vi "Map.vi"() -> ()   [LabVIEW 2015]
uses:
  Robot.ctl
  Instruction.ctl
  class/Car.lvclass
  class/Instruction.lvclass
  class/MovementInstruction.lvclass
  class/TurnInstruction.lvclass
  class/StopInstruction.lvclass
  <vilib>/rvi/interface/nirviReadWriteControl/nirviReadWriteControl.xnode
  class/SonarSensor.lvclass
  <vilib>/rvi/interface/nirviCloseFPGA/nirviCloseFPGA.xnode
  <vilib>/rvi/interface/nirviOpenFPGA/nirviOpenFPGA.xnode
  NiFpgaLv.dll
  <vilib>/Utility/error.llb/Error Cluster From Error Code.vi
  <vilib>/rvi/interface/Simulation/niFpgaSimulationCallBeginRW.vi
  <vilib>/rvi/errors/niLvFpgaAdjustHostInterfaceError.vi
  <vilib>/FPGAPlugInAG/Dynamic/niLvFpga_Close_Dynamic.vi
  FPGA Bitfiles/Milestone4_FPGATarget_FPGAReadSonars_MhsUmP2nS8s.lvbitx
  physical_robot/FPGA Read Sonars.vi
  <vilib>/FPGAPlugInAG/myRIO-1900/niLvFpga_Open_myRIO-1900.vi
  <vilib>/rvi/interface/common/dynamic/niFpgaDynamicAddResources.vi
panel:
  out "millisecond timer value":u32
  out "x .or. y?":bool
  out "Sim Robot Properties":T1={"Position"=[0.0, 0.0], "Size"=50.0, "Facing"=0.0, "Movement Ratios"=[0.0, -1.0], "Wheel Angle"=0.0}
  in  "Robot Properties":T1={"Position"=[500.0, 500.0], "Size"=33.0, "Facing"=0.0, "Movement Ratios"=[0.0, -1.0], "Wheel Angle"=0.0}
  out "Completed":bool
  out "Instruction Number":i32
  in  "Instructions":T2[](array[typedef])=[{"Type"="Movement", "Variable A"=30.0, "Variable B"=300.0, "Variable C"=0.0}, {"Type"="Turn", "Variable A"=30.0, "Variable B"=20.0, "Variable C"=90.0}, {"Type"="Movement", "Variable A"=30.0, "Variable B"=250.0, "Variable C"=0.0}, {"Type"="Turn", "Variable A"=30.0, "Variable B"=20.0, "Variable C"=90.0}, {"Type"="Movement", "Variable A"=30.0, "Variable B"=300.0, "Variable C"=0.0}, {"Type"="Stop", "Variable A"=3000.0, "Variable B"=0.0, "Variable C"=0.0}, {"Type"="Movement", "Variable A"=30.0, "Variable B"=200.0, "Variable C"=0.0}, {"Type"="Turn", "Variable A"=30.0, "Variable B"=-20.0, "Variable C"=90.0}, {"Type"="Movement", "Variable A"=30.0, "Variable B"=250.0, "Variable C"=0.0}, {"Type"="Turn", "Variable A"=30.0, "Variable B"=-20.0, "Variable C"=90.0}, {"Type"="Movement", "Variable A"=30.0, "Variable B"=300.0, "Variable C"=0.0}, {"Type"="Stop", "Variable A"=3000.0, "Variable B"=0.0, "Variable C"=0.0}]
  out "Robot Properties Output":T1
  in  "stop":bool
  in  "Obstacles":dbl[][](array[numeric])=[[100.0, 100.0, 420.0, 110.0], [100.0, 100.0, 110.0, 300.0], [100.0, 290.0, 420.0, 300.0], [410.0, 100.0, 420.0, 300.0], [205.0, 190.0, 215.0, 300.0], [305.0, 190.0, 315.0, 300.0]]
  out "2D Picture":picture
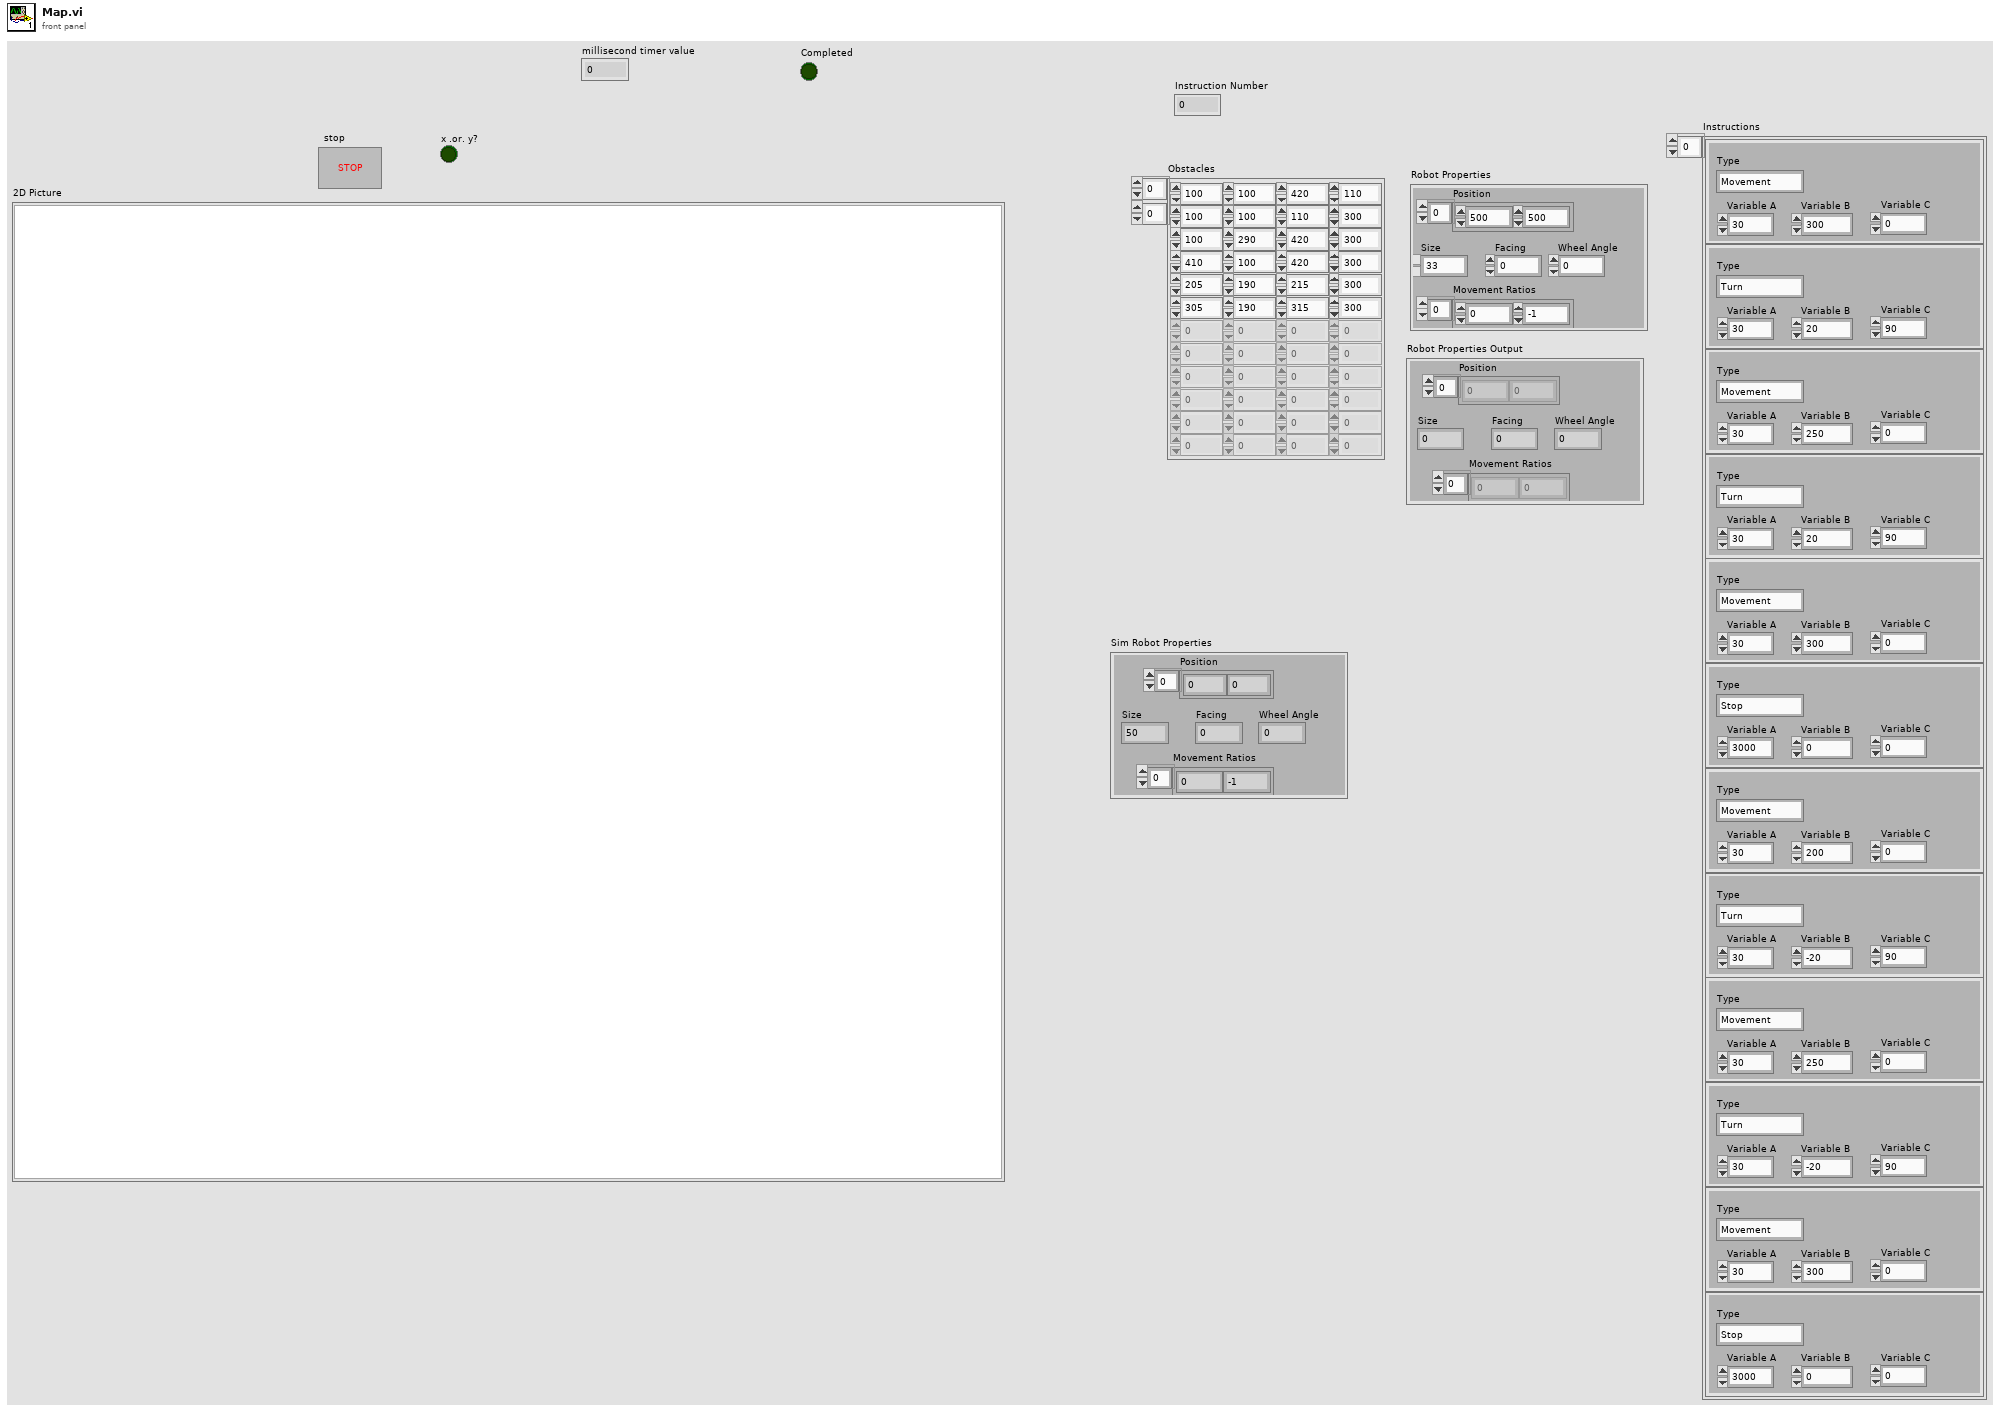
[diagram p1: front panel]
types:
  T1 = typedef "Robot.ctl" = cluster{"Position":dbl[], "Size":dbl, "Facing":dbl, "Movement Ratios":dbl[], "Wheel Angle":dbl}
  T2 = typedef "Instruction.ctl" = cluster{"Type":string, "Variable A":dbl, "Variable B":dbl, "Variable C":dbl}
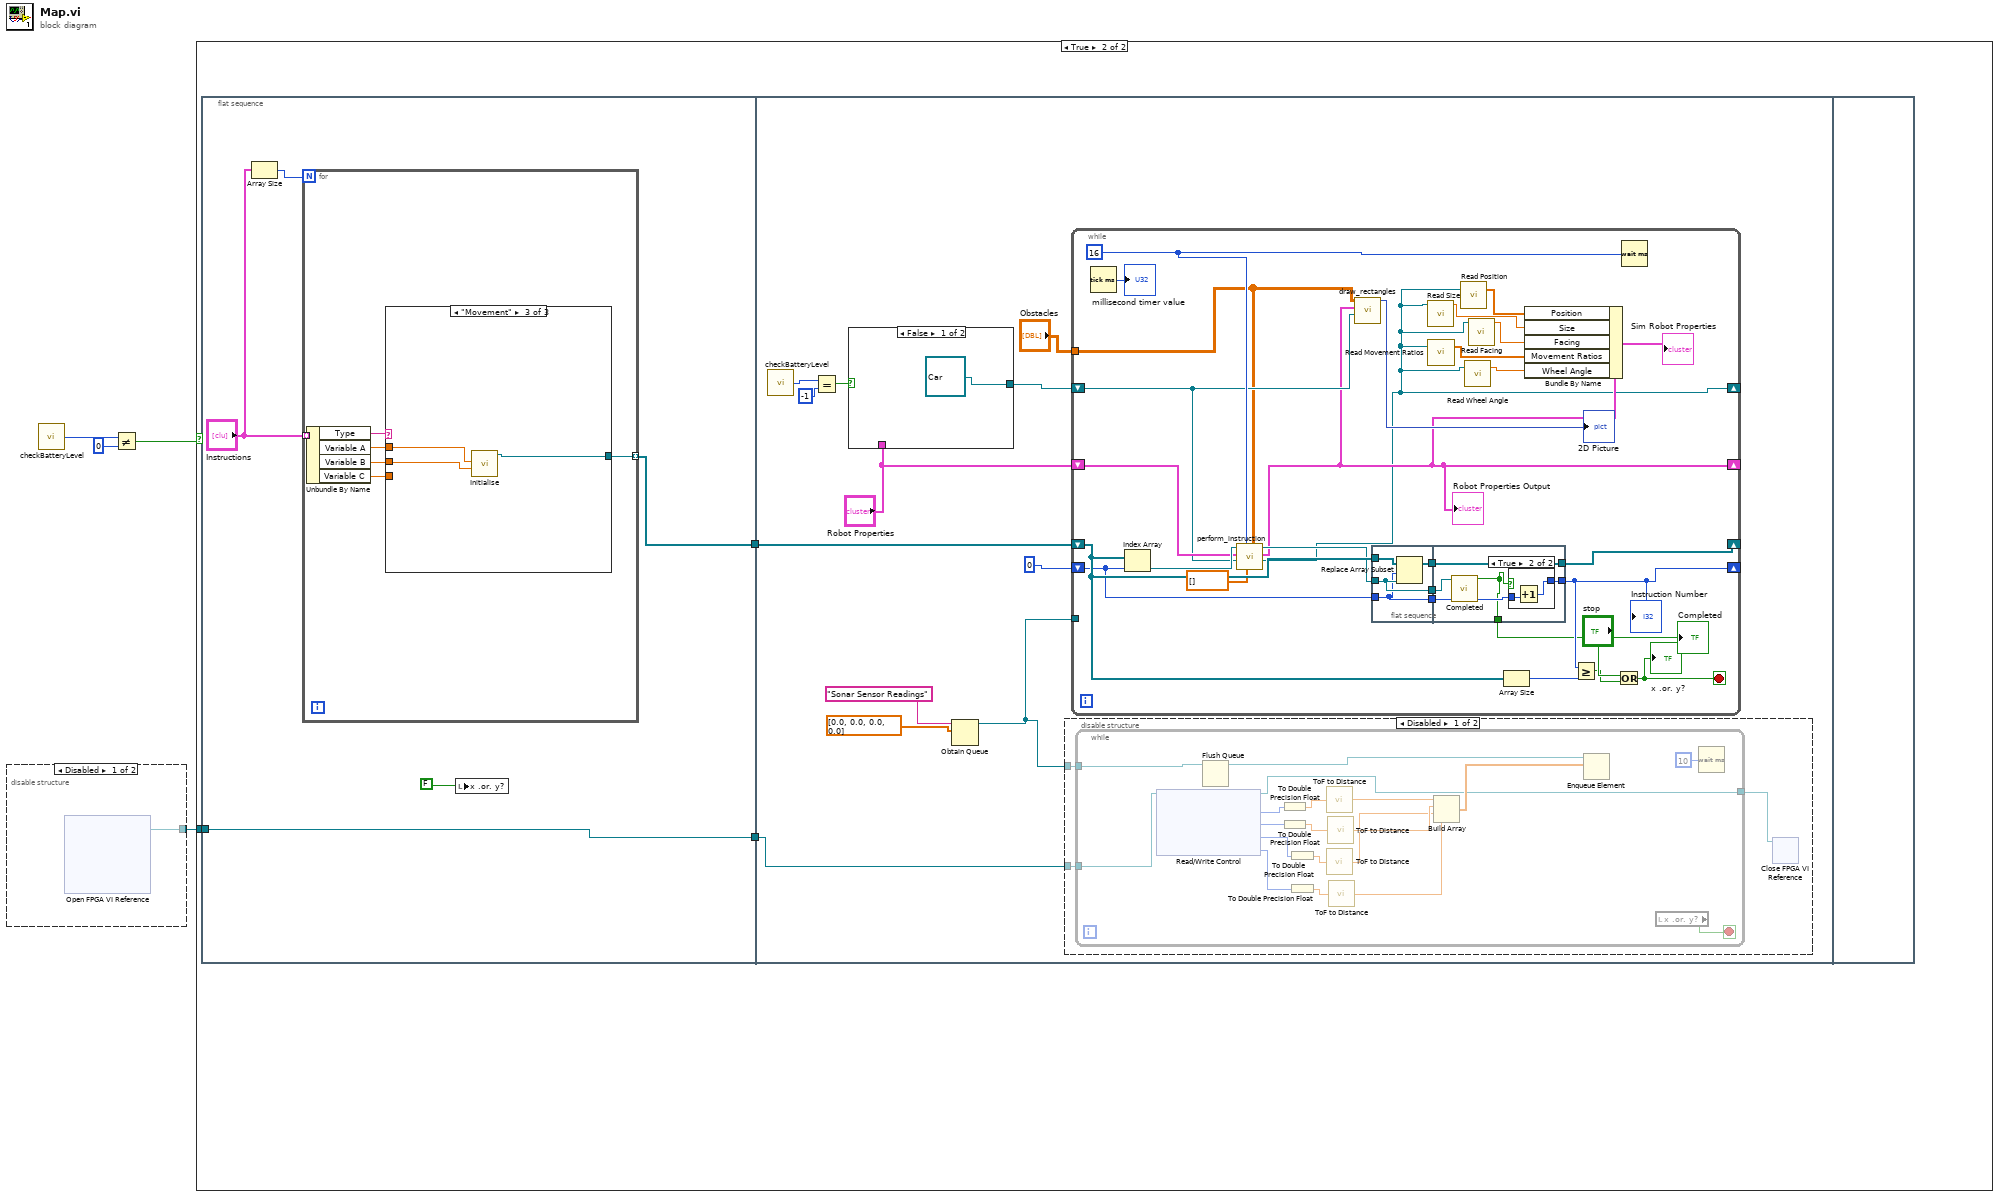
[diagram p0: block diagram]
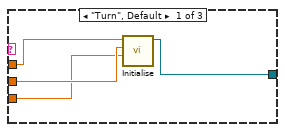
[diagram p4: hidden frame]
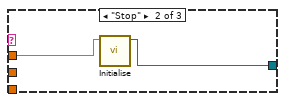
[diagram p5: hidden frame]
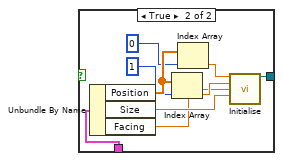
[diagram p7: hidden frame]
diagram:
  n1 = disable-structure shown="Disabled" {
    disable-tunnel: [w5 _] -> w1
    frame Disabled {
      n2 = xnode "Open FPGA VI Reference"() -> ("FPGA VI Reference Out"=w5:refnum<k20>)  [unwired: 2 in, 1 out]
    }
    frame Enabled {
    }
  }
  n3 = call "checkBatteryLevel.vi"() -> ("Battery State"=w4:i32)
  n4 = Not Equal?(x=w4, y=0) -> (x != y?=w2:bool)
  n5 = case shown="True" w2 {
    tunnel: w1 -> [_ w6]
    frame False {
    }
    frame True {
      n6 = flat-sequence {
        tunnel: [w9] -> w8
        tunnel: [w11] -> w7
        tunnel: w6 -> [w11]
        tunnel: w8 -> [w39]
        tunnel: w7 -> [w30]
        frame #0 {
          n7 = Array Size(array="Instructions") -> (size(s)=w13:i32)
          n8 = for {
            N: w13 -> [_]
            tunnel: "Instructions" -> [w19] mode=indexing
            tunnel: [w17] -> w9 mode=indexing
            n9 = Unbundle By Name(w19) -> ("Type"=w18:string, "Variable A"=w16:dbl, "Variable B"=w15:dbl, "Variable C"=w14:dbl)
            n10 = case shown="\"Movement\"" w18 {
              tunnel: [w20 w24 w28] -> w17
              tunnel: w16 -> [w23 w25 w27]
              tunnel: w15 -> [w22 _ w26]
              tunnel: w14 -> [w21 _ _]
              frame "Turn", Default {
                n11 = call "Initialise.vi"("Angle to Turn"=w21, "Wheel Angle"=w22, "Speed"=w23) -> ("TurnInstruction.lvclass"=w20:refnum<class "TurnInstruction.lvclass">)  [unwired: 7 in, 1 out]
              }
              frame "Stop" {
                n12 = call "Initialise.vi"("Time to wait"=w25) -> ("StopInstruction out"=w24:refnum<class "StopInstruction.lvclass">)  [unwired: 9 in, 1 out]
              }
              frame "Movement" {
                n13 = call "Initialise.vi"("Distance"=w26, "Speed"=w27) -> ("MovementInstruction.lvclass"=w28:refnum<class "MovementInstruction.lvclass">)  [unwired: 8 in, 1 out]
              }
            }
          }
          n14 = local write "x .or. y?"(FALSE) -> ()
        }
        frame #1 {
          n15 = call "checkBatteryLevel.vi"() -> ("Battery State"=w35:i32)
          n16 = Equal?(x=w35, y=-1) -> (x = y?=w33:bool)
          n17 = case shown="False" w33 {
            tunnel: "Robot Properties" -> [_ w72]
            tunnel: [refnum<class "Car.lvclass"> refnum ("Car.lvclass") w64] -> w36
            frame False {
            }
            frame True {
              n18 = Unbundle By Name(w72) -> ("Position"=w70:dbl[], "Size"=w66:dbl, "Facing"=w65:dbl)
              n19 = Index Array(array=w70, index=1) -> (element=w69:dbl)
              n20 = Index Array(array=w70, index=0) -> (element=w71:dbl)
              n21 = call "Initialise.vi"("X"=w71, "Y"=w69, "Facing"=w65, "Size"=w66) -> ("Car.lvclass"=w64:refnum<class "Car.lvclass">)  [unwired: 10 in, 1 out]
            }
          }
          n22 = Obtain Queue(name (unnamed)="Sonar Sensor Readings", element data type=dbl[] [0.0, 0.0, 0.0, 0.0]) -> (queue out=w29:refnum<queue>)  [unwired: 3 in, 2 out]
          n23 = disable-structure shown="Disabled" {
            disable-tunnel: w30 -> [w43 _]
            disable-tunnel: w29 -> [w42 _]
            frame Disabled {
              n24 = while {
                tunnel: w43 -> [w50]
                tunnel: w42 -> [w47]
                tunnel: [w44] -> w41
                stop <- w48 stop-if-true
                n25 = xnode "Read/Write Control"("FPGA VI Reference In"=w50) -> ("FPGA VI Reference Out"=w44:refnum<k20>, "Time of Flight Front"=w61:u32, "Time of Flight Right"=w60:u32, "Time of Flight Back"=w58:u32, "Time of Flight Left"=w56:u32)  [unwired: 1 in, 1 out]
                n26 = Flush Queue(queue=w47) -> (queue out=w45:refnum<queue>)  [unwired: 1 in, 2 out]
                n27 = To Double Precision Float(number=w61) -> (double precision float=w62:dbl)
                n28 = To Double Precision Float(number=w60) -> (double precision float=w59:dbl)
                n29 = To Double Precision Float(number=w58) -> (double precision float=w57:dbl)
                n30 = To Double Precision Float(number=w56) -> (double precision float=w55:dbl)
                n31 = call "ToF to Distance.vi"("Time of Flight"=w62) -> ("Distance"=w54:dbl)
                n32 = call "ToF to Distance.vi"("Time of Flight"=w57) -> ("Distance"=w52:dbl)
                n33 = call "ToF to Distance.vi"("Time of Flight"=w59) -> ("Distance"=w53:dbl)
                n34 = call "ToF to Distance.vi"("Time of Flight"=w55) -> ("Distance"=w51:dbl)
                n35 = Build Array(w54, w53, w52, w51) -> (w46:dbl[])
                n36 = Enqueue Element(queue=w45, element=w46) -> ()  [unwired: 2 in, 3 out]
                n37 = local read "x .or. y?"() -> (w48:bool)
                n38 = Wait (ms)(milliseconds to wait=u32 10) -> ()  [unwired: 1 out]
              }
              n39 = xnode "Close FPGA VI Reference"("FPGA VI Reference In"=w41) -> ()  [unwired: 1 in, 1 out]
            }
            frame Enabled {
            }
          }
          n40 = while {
            tunnel: "Obstacles" -> [w76]
            shift-right: [w84] -> _
            shift-left: "Robot Properties" -> [w87]
            shift-right: [w91] -> _
            shift-left: 0 -> [w96]
            shift-right: [w95] -> _
            shift-left: w39 -> [w97]
            shift-right: [w77] -> _
            shift-left: w36 -> [w85]
            tunnel: w29 -> [_]
            stop <- w75 stop-if-true
            w86 = u32 16 ("milliseconds to wait")
            n41 = Tick Count (ms)() -> (millisecond timer value=→"millisecond timer value":u32)
            n42 = Index Array(array=w97, index=w96) -> (element=w88:refnum<class "Instruction.lvclass">)
            n43 = call "perform_instruction.vi"("Obstacles"=w76, "Sonar Readings"=dbl[] [], "Time Since Last Instruction"=w86, "Car.lvclass"=w85, "Robot Properties"=w87, "Instruction.lvclass"=w88) -> ("Car.lvclass 2"=w77:refnum<class "Car.lvclass">, "Robot Properties 2"=w84:T1, "Instruction.lvclass 2"=w89:refnum<class "Instruction.lvclass">)  [unwired: 2 in, 1 out]
            "Robot Properties Output" <- w84
            n44 = call "draw_rectangles.vi"("Rectangle Array"=w76, "Robot Properties"=w84, "Sim Car.lvclass"=w85) -> ("Map Picture"=→"2D Picture":picture)  [unwired: 7 in]
            n45 = flat-sequence {
              tunnel: w89 -> [w103]
              tunnel: w97 -> [w105]
              tunnel: w96 -> [w102]
              tunnel: [w104] -> w94
              tunnel: [w103] -> w93
              tunnel: [w102] -> w92
              tunnel: [w110] -> w95
              tunnel: w94 -> [w110]
              tunnel: w93 -> [w107]
              tunnel: w92 -> [w109]
              tunnel: [w108] -> w91
              tunnel: [w106] -> w90
              frame #0 {
                n46 = Replace Array Subset(array=w105, new element=w103, index=w102) -> (w104:refnum<class "Instruction.lvclass">[])
              }
              frame #1 {
                n47 = call-dynamic "Completed.vi"("Instruction in"=w107) -> ("Completed"=w106:bool)  [unwired: 9 in, 1 out]
                n48 = case shown="True" w106 {
                  tunnel: w109 -> [w111 w113]
                  tunnel: [w111 w112] -> w108
                  frame False {
                  }
                  frame True {
                    n49 = Increment(x=w113) -> (x+1=w112:i32)
                  }
                }
              }
            }
            n50 = call "Read Size.vi"("Car.lvclass"=w77) -> ("Size"=w81:dbl)  [unwired: 9 in, 1 out]
            n51 = call "Read Movement Ratios.vi"("Car.lvclass"=w77) -> ("Array"=w79:dbl[])  [unwired: 1 in, 1 out]
            n52 = call "Read Position.vi"("Car.lvclass"=w77) -> ("Position"=w82:dbl[])  [unwired: 1 in, 1 out]
            n53 = call "Read Wheel Angle.vi"("Car.lvclass"=w77) -> ("Wheel Angle"=w78:dbl)  [unwired: 1 in, 1 out]
            n54 = call "Read Facing.vi"("Car.lvclass"=w77) -> ("Facing"=w80:dbl)  [unwired: 9 in, 1 out]
            n55 = Array Size(array=w97) -> (size(s)=w100:i32)
            n56 = Bundle By Name(cluster=w84, "Position"=w82, "Size"=w81, "Facing"=w80, "Movement Ratios"=w79, "Wheel Angle"=w78) -> (→"Sim Robot Properties":T1)
            n57 = Greater Or Equal?(x=w91, y=w100) -> (x >= y?=w98:bool)
            n58 = Or(x="stop", y=w98) -> (x .or. y?=w75:bool)
            "x .or. y?" <- w75
            n59 = Wait (ms)(milliseconds to wait=w86) -> ()  [unwired: 1 out]
            "Instruction Number" <- w91
            "Completed" <- w90
          }
        }
        frame #2 {
        }
      }
    }
  }
